vi "oa_Time Positions Linear Backward Extrapolation.vi"(5 "number of points":i32=4, 7 "reset? (T)":bool=TRUE, 8 "positions [s]":dbl[](array[numeric]), 9 "filter length":i32, 10 "dr":dbl=1.0 format="%.2p", 11 "r0":dbl format="%.2p") -> (0 "extraploated positions [s]":dbl[](array[numeric]), 1 "dr out":dbl=1.0 format="%.2p", 2 "new r0":dbl format="%.2p")   [LabVIEW 2017, in "SoundVib_OAUtility.lvlib"]
uses:
  <vilib>/addons/Sound and Vibration/Order Analysis/Utility/SoundVib_OAUtility.lvlib
  <vilib>/Analysis/NI_AALBase.lvlib
  <vilib>/Analysis/NI_AALPro.lvlib
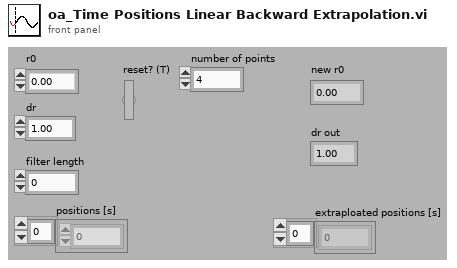
[diagram p1: front panel]
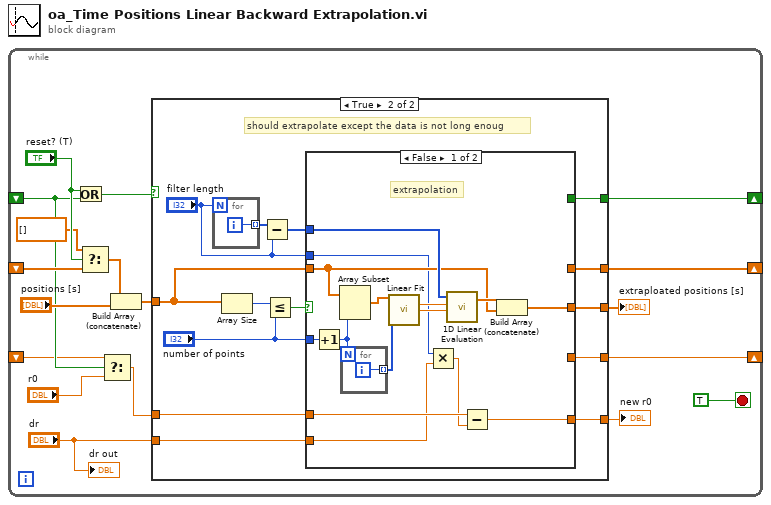
[diagram p0: block diagram]
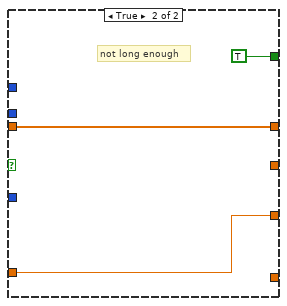
[diagram p3: hidden frame]
diagram:
  n1 = while {
    shift-right: [w18] -> _
    shift-left: _ -> [w6]
    shift-right: [w14] -> _
    shift-left: _ -> [w11]
    shift-right: [w7] -> _
    shift-left: _ -> [w5]
    stop <- TRUE stop-if-true
    n2 = Or(x="reset? (T)", y=w6) -> (x .or. y?=w2:bool)
    n3 = Select(t=dbl[] [], s="reset? (T)", f=w11) -> (s? t:f=w12:dbl[])
    n4 = Select(t=w5, s=w6, f="r0") -> (s? t:f=w3:dbl)
    n5 = Build Array (concatenate)(w12, "positions [s]") -> (w13:dbl[])
    n6 = case shown="True" w2 {
      tunnel: [_ w29] -> w18
      tunnel: w13 -> [w20 w31]
      tunnel: [w20 w32] -> w15
      tunnel: [_ w30] -> w14
      tunnel: [w19 w24] -> w8
      tunnel: w3 -> [w19 w26]
      tunnel: [_ w23] -> w7
      tunnel: "dr" -> [_ w21]
      frame False {
      }
      frame True {
        # "should extrapolate except the data is not long enoug"
        n7 = for {
          N: "filter length" -> [_]
          tunnel: [w35] -> w28 mode=indexing
          i -> [w35]
        }
        n8 = Array Size(array=w31) -> (size(s)=w34:i32)
        n9 = Subtract(x=w28, y="filter length") -> (x-y=w27:i32[])
        n10 = Less Or Equal?(x=w34, y="number of points") -> (x <= y?=w33:bool)
        n11 = case shown="False" w33 {
          tunnel: [w44 _] -> w32
          tunnel: [_ w54] -> w30
          tunnel: w31 -> [w45 w54]
          tunnel: [_ TRUE] -> w29
          tunnel: w27 -> [w47 _]
          tunnel: w26 -> [w42 w52]
          tunnel: "filter length" -> [w43 _]
          tunnel: [w40 _] -> w24
          tunnel: [_ w52] -> w23
          tunnel: "number of points" -> [w39 _]
          tunnel: w21 -> [w38 _]
          frame False {
            # "extrapolation"
            n12 = Increment(x=w39) -> (x+1=w36:i32)
            n13 = Array Subset(array=w45, length=w36) -> (w50:dbl[])  [unwired: 1 in]
            n14 = for {
              N: w36 -> [_]
              tunnel: [w51] -> w37 mode=indexing
              i -> [w51]
            }
            n15 = call <vilib>:"Linear Fit.vi"("Y"=w50, "X"=w37) -> ("slope"=w49:dbl, "intercept"=w48:dbl)  [unwired: 9 in, 3 out]
            n16 = Multiply(x=w43, y=w38) -> (x*y=w41:dbl)
            n17 = call <vilib>:"1D Linear Evaluation.vi"("offset"=w48, "scale"=w49, "X"=w47) -> ("Y[i]=X[i]*a+b"=w46:dbl[])  [unwired: 1 out]
            n18 = Subtract(x=w42, y=w41) -> (x-y=w40:dbl)
            n19 = Build Array (concatenate)(w46, w45) -> (w44:dbl[])
          }
          frame True {
            # "not long enough"
          }
        }
      }
    }
    "extraploated positions [s]" <- w15
    "new r0" <- w8
    "dr out" <- "dr"
  }
